vi "Div-Volt.vi"(0 "V_S":dbl, 1 "R2":dbl, 2 "R1":dbl) -> (3 "V_S  /  R_EQ":dbl, 4 "R_EQ":dbl, 5 "I2":dbl, 6 "I1":dbl)   [LabVIEW 2010]
doc: "Calculate voltage at individual series resistors (R1, R2) within a containing circuit, provided voltage (V_S) of the containing circuit\n\nVn = V_s * ( Rn / R_EQ )"
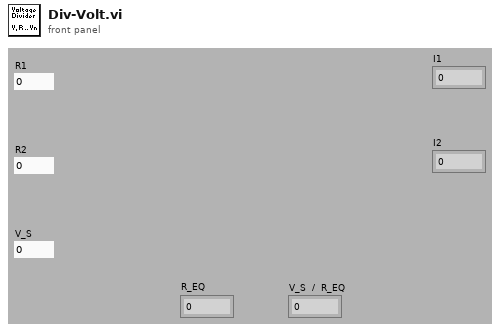
[diagram p1: front panel]
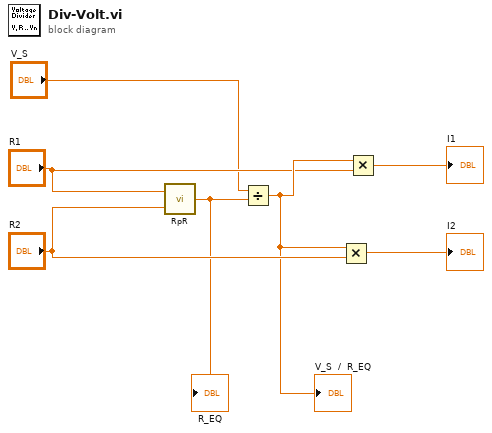
[diagram p0: block diagram]
diagram:
  n1 = call "RpR.vi"("R2"="R2", "R1"="R1") -> ("R1 // R2"=w1:dbl)  [unwired: 2 out]
  "R_EQ" <- w1
  n2 = Divide(x="V_S", y=w1) -> (x/y=w4:dbl)
  "V_S  /  R_EQ" <- w4
  n3 = Multiply(x=w4, y="R2") -> (x*y=→"I2":dbl)
  n4 = Multiply(x=w4, y="R1") -> (x*y=→"I1":dbl)
